vi "Shooter Ready.vi"(9 "percent err":dbl, 10 "flywheel speed":dbl, 11 "target speed":dbl) -> (3 "up to speed?":bool)   [LabVIEW 2020]
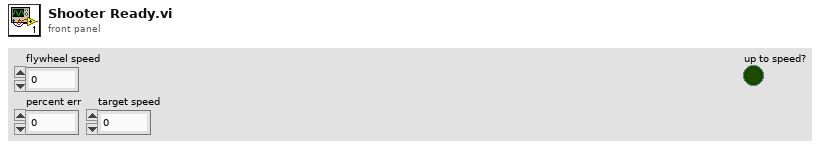
[diagram p1: front panel]
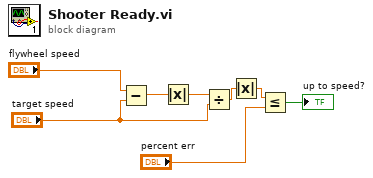
[diagram p0: block diagram]
diagram:
  n1 = Subtract(x="flywheel speed", y="target speed") -> (x-y=w7:dbl)
  n2 = Absolute Value(x=w7) -> (abs(x)=w6:dbl)
  n3 = Divide(x=w6, y="target speed") -> (x/y=w2:dbl)
  n4 = Absolute Value(x=w2) -> (abs(x)=w1:dbl)
  n5 = Less Or Equal?(x=w1, y="percent err") -> (x <= y?=→"up to speed?":bool)
